vi "RT Loop - DI Changed.vi"(11 "Message Queue":refnum<queue>) -> ()   [LabVIEW 2018]
doc: "This Control Loop VI performs control calculations of diverter line (DL) rotation."
uses:
  Support/Message Queue/Message Cluster.ctl
  Support/Message Queue/Message.ctl
  <vilib>/Platform/TimedLoop/XDataNode/timing_clust.ctl
  <vilib>/Platform/TimedLoop/XDataNode/nitl_modes.ctl
  <vilib>/Platform/TimedLoop/XDataNode/wakeup.ctl
  <vilib>/Platform/TimedLoop/XDataNode/loadnilvce.vi
  Globals/Global - RT Channels.vi
  <vilib>/Platform/TimedLoop/XDataNode/XDataNode.xnode
  <vilib>/Platform/TimedLoop/XDataNode/XDNodeRunTimeDep.lvlib
  support/Message Queue/Message Queue.lvlib
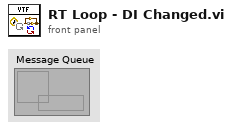
[diagram p1: front panel]
types:
  T1 = typedef "XDNodeRunTimeDep.lvlib/timing_clust.ctl" = cluster{"Expected End [f-1]":u64, "Actual End [f-1]":u64, "Finished Late? [f-1]":bool, "Expected End [i-1]":u64, "Actual End [i-1]":u64, "Finished Late? [i-1]":bool, "Expected Start [i]":u64, "Actual Start [i]":u64, "Expected Start [f]":u64, "Actual Start [f]":u64, "Source Name":string, "Structure Name":string, "Period":i64, "Deadline":i64, "Offset":i64, "Start":i64, "Priority":i32, "Timeout":i32, "Mode":T2, "Wakeup Reason":T3, "Error":errorcluster, "Source Type":string, "Secondary Source Type":string, "Global End Time":u64, "Global Start Time":u64, "Frame Duration":u64, "Iteration Duration":u64, "Assigned CPU":i32, "I/O Scan Engine Mode":u32}
  T2 = typedef "XDNodeRunTimeDep.lvlib/nitl_modes.ctl" = enum32{"No Change", "Process missed periods, maintain original phase", "Discard missed periods, maintain original phase", "Process missed periods, ignore original phase", "Discard missed periods, ignore original phase"}
  T3 = typedef "XDNodeRunTimeDep.lvlib/wakeup.ctl" = enum32{"Normal", "Aborted", "Asynchronous wakeup", "Timing source error", "Timed loop error", "Timeout"}
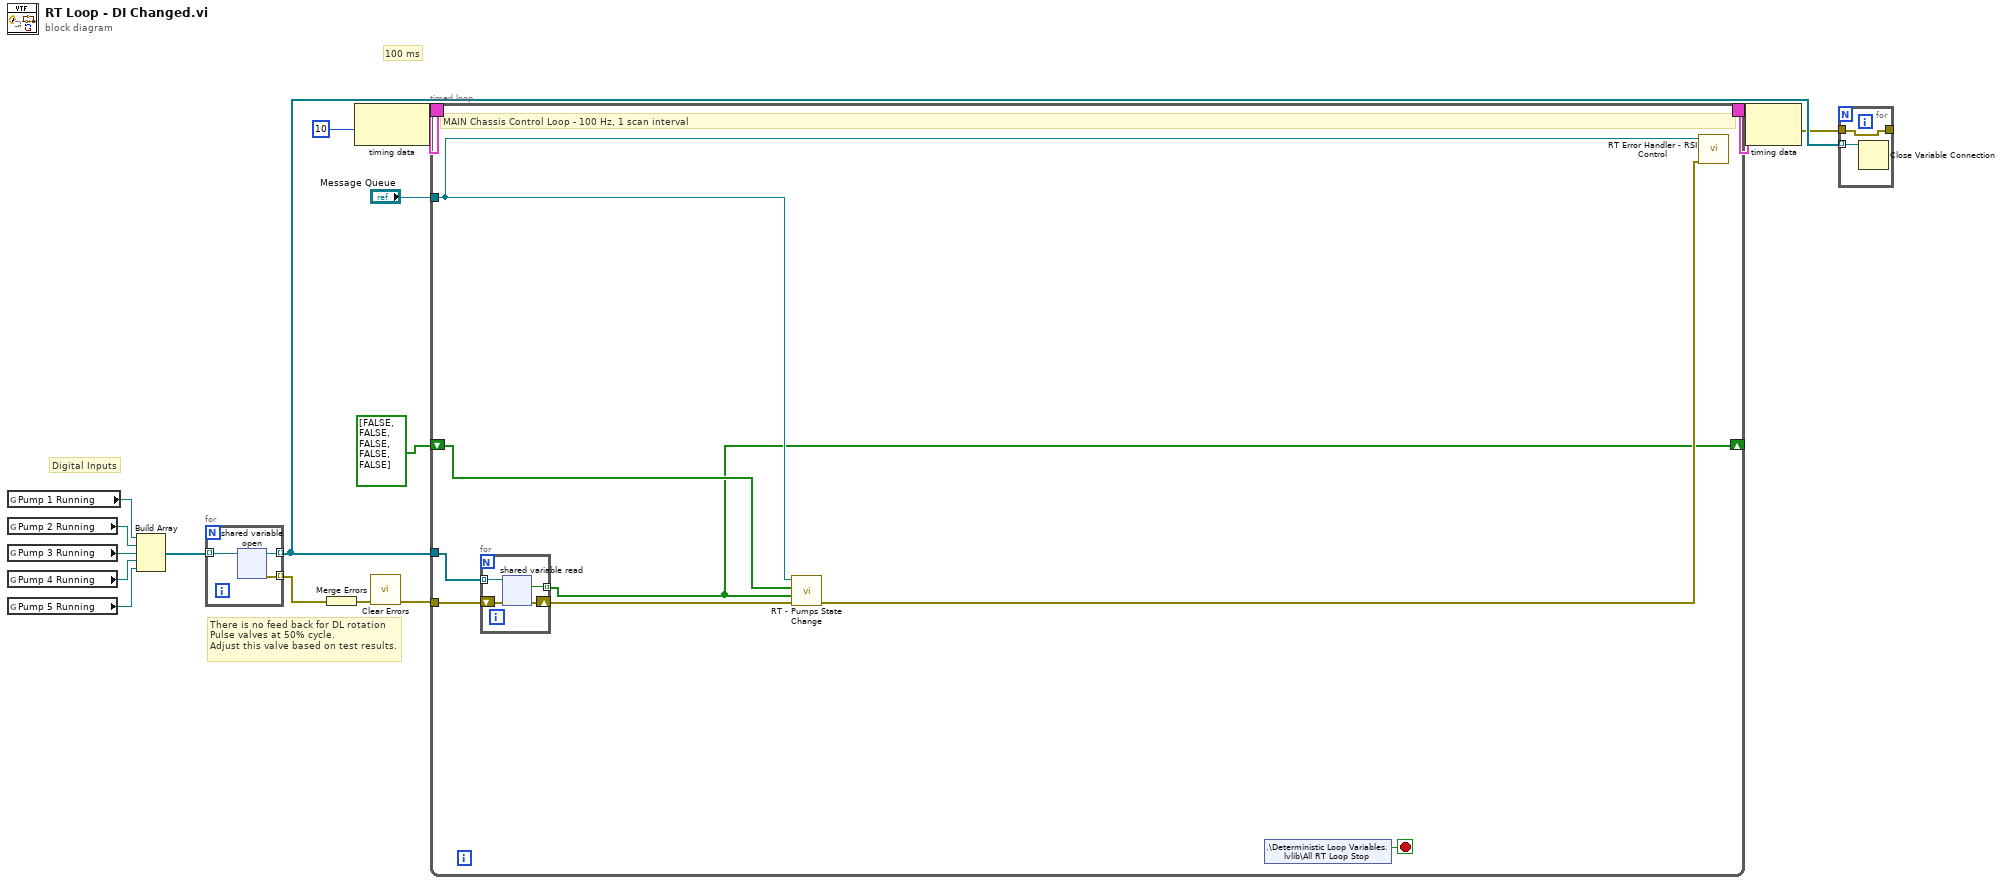
[diagram p0: block diagram]
diagram:
  # "100 ms"
  # "Digital Inputs"
  # "There is no feed back for DL rotation\nPulse valves at 50% cycle. \nAdjust this valve based on test results."
  n1 = global read "Global - RT Channels.vi" "Pump 1 Running"() -> (w3:refnum<k21>)
  n2 = global read "Global - RT Channels.vi" "Pump 2 Running"() -> (w4:refnum<k21>)
  n3 = global read "Global - RT Channels.vi" "Pump 3 Running"() -> (w5:refnum<k21>)
  n4 = global read "Global - RT Channels.vi" "Pump 4 Running"() -> (w6:refnum<k21>)
  n5 = global read "Global - RT Channels.vi" "Pump 5 Running"() -> (w7:refnum<k21>)
  n6 = Build Array(w3, w4, w5, w6, w7) -> (w2:refnum<k21>[])
  n7 = for {
    tunnel: w2 -> [w19] mode=indexing
    tunnel: [w18] -> w11 mode=indexing
    tunnel: [w17] -> w8 mode=indexing
    n8 = shared-variable-open(w19) -> (w18:refnum<k21>, w17:errorcluster)  [unwired: 1 in]
  }
  n9 = Merge Errors(w8) -> (w9:errorcluster)
  n10 = node-c288(i64 10 ("Period")) -> (w16:T1)
  n11 = call <vilib>:"Clear Errors.vi"("error in (no error)"=w9) -> ("error out"=w12:errorcluster)  [unwired: 5 in, 1 out]
  n12 = timed-loop {
    timing: w16 -> [_]
    timing-out: [_] -> w15
    tunnel: "Message Queue" -> [w24]
    tunnel: w12 -> [w25]
    tunnel: w11 -> [w26]
    shift-right: [w20] -> _
    shift-left: bool[] [FALSE, FALSE, FALSE, FALSE, FALSE] ("Pumps State In") -> [w22]
    stop <- w27 stop-if-true
    # "MAIN Chassis Control Loop - 100 Hz, 1 scan interval"
    n13 = for {
      tunnel: w26 -> [w30] mode=indexing
      shift-right: [w31] -> w21
      shift-left: w25 -> [w29]
      tunnel: [w28] -> w20 mode=indexing
      n14 = shared-variable-read(w30, w29) -> (w31:errorcluster, w28:bool)  [unwired: 1 out]
    }
    n15 = call "RT - Pumps State Change.vi"("error in"=w21, "Pumps State"=w20, "Pumps State In"=w22, "Queue in"=w24) -> ("error out"=w23:errorcluster)  [unwired: 7 in]
    n16 = shared-variable ".\\Deterministic Loop Variables.lvlib\\All RT Loop Stop"() -> (w27:bool)  [unwired: 1 in, 1 out]
    n17 = call "RT Error Handler - RSI Control.vi"("error in (no error)"=w23, "Message Queue"=w24) -> ()  [unwired: 8 in, 2 out]
  }
  n18 = node-c288(w15) -> (w10:errorcluster)
  n19 = for {
    tunnel: w10 -> [w34]
    tunnel: w11 -> [w35] mode=indexing
    tunnel: [w34] -> _
    n20 = Close Variable Connection(11:w35) -> ()  [unwired: 1 in, 1 out]
  }
